vi "Check Previous Error.vi"(8 "error in (no error)":errorcluster, 11 "VISA resource name in":refnum<visa-resource-name>) -> (0 "error out":errorcluster, 3 "VISA resource name":refnum<visa-resource-name>)   [LabVIEW 2024, in "CTIPicoVISA.lvlib"]
uses:
  CTIPicoVISA.lvlib
  <vilib>/Utility/error.llb/whitespace.ctl
  <vilib>/Utility/error.llb/Trim Whitespace One-Sided.vi
  <vilib>/Utility/error.llb/Error Cluster From Error Code.vi
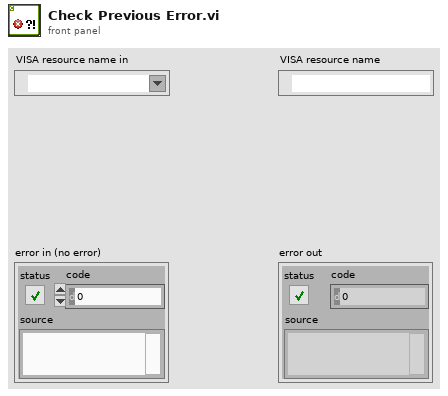
[diagram p1: front panel]
types:
  T1 = typedef "whitespace.ctl" = u16
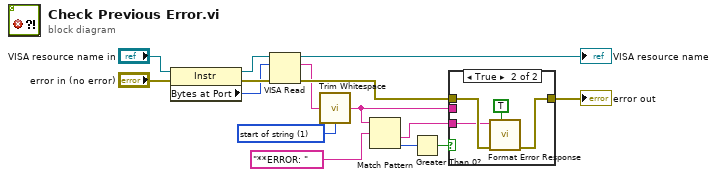
[diagram p0: block diagram]
diagram:
  w7 = T1 1 items=["both", "start of string", "end of string"] ("location (both)")
  n1 = property class="Instr"(reference="VISA resource name in", error in="error in (no error)") -> (reference out=w11:refnum<visa-resource-name>, error out=w14:errorcluster, "Bytes at Port"=w10:u32)
  n2 = VISA Read(VISA resource name=w11, byte count=w10, error in (no error)=w14) -> (VISA resource name out=→"VISA resource name":refnum<visa-resource-name>, read buffer=w8:string, error out=w15:errorcluster)  [unwired: 1 out]
  n3 = call <vilib>:"Trim Whitespace.vi"("string"=w8, "location (both)"=w7) -> ("trimmed string"=w5:string)
  n4 = Match Pattern(string=w5, regular expression="**ERROR: " ("x")) -> (after substring=w4:string, offset past match=w3:i32)  [unwired: 1 in, 2 out]
  n5 = Greater Than 0?(x=w3) -> (x > 0?=w2:bool)
  n6 = case shown="True" w2 {
    tunnel: w15 -> [w16 w20]
    tunnel: w5 -> [_ _]
    tunnel: w4 -> [_ w19]
    tunnel: [w16 w17] -> w1
    frame False {
    }
    frame True {
      n7 = call "Format Error Response.vi"("show call chain? (False)"=TRUE, "error in (no error)"=w20, "Error Response"=w19) -> ("error out"=w17:errorcluster)  [unwired: 8 in]
    }
  }
  "error out" <- w1
